vi "Impulsator.vi"(1 "PV":dbl format="%#.1g", 2 "upper limit":dbl=100.0 format="%#_13g", 4 "Initialise":bool) -> (0 "Y":bool)   [LabVIEW 2019, in "Userlib.lvlib"]
uses:
  Userlib.lvlib
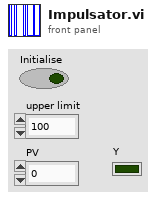
[diagram p1: front panel]
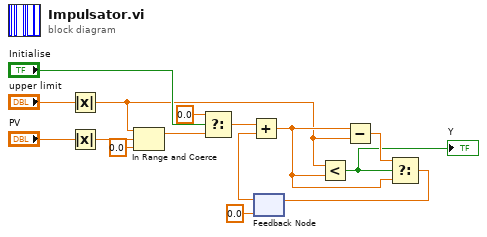
[diagram p0: block diagram]
diagram:
  n1 = Absolute Value(x="upper limit") -> (abs(x)=w3:dbl)
  n2 = Absolute Value(x="PV") -> (abs(x)=w1:dbl)
  n3 = In Range and Coerce(upper limit=w3, x=w1, lower limit=0.0) -> (coerced(x)=w10:dbl)  [unwired: 1 out]
  n4 = Select(t=0.0, s="Initialise", f=w10) -> (s? t:f=w13:dbl)
  n5 = feedback #1(0.0) -> (w15:dbl)
  n6 = Add(x=w13, y=w15) -> (x+y=w7:dbl)
  n7 = Less?(x=w3, y=w7) -> (x < y?=w5:bool)
  "Y" <- w5
  n8 = Subtract(x=w7, y=w3) -> (x-y=w8:dbl)
  n9 = Select(t=w8, s=w5, f=w7) -> (s? t:f=w6:dbl)
  n10 = feedback-in #1(w6) -> ()
